vi "PID Table (Auto).vi"(6 "Ziegler-Nichlos Speed":u16(ring) items=["Fast", "Normal", "Slow"], 7 "Type of Controller":u16(ring) items=["P", "PI", "PID"], 8 "dT":dbl, 9 "Dead Time (L)":dbl, 10 "Time Constant (T)":dbl, 11 "Plant Gain (K)":dbl) -> (1 "Derivative Time (Td)":dbl, 2 "Integral Time (Ti)":dbl, 3 "Proportional Gain (Kp)":dbl)   [LabVIEW 2020, in "NI_PID_autopid.lvlib"]
uses:
  <vilib>/addons/control/pid/NI_PID_autopid.lvlib
  <vilib>/addons/control/pid/NI_PID_pid.lvlib
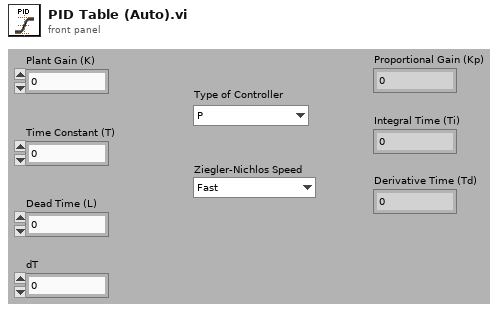
[diagram p1: front panel]
types:
  T1 = enum16{"Academic (Standard)", "Parallel", "Series"}
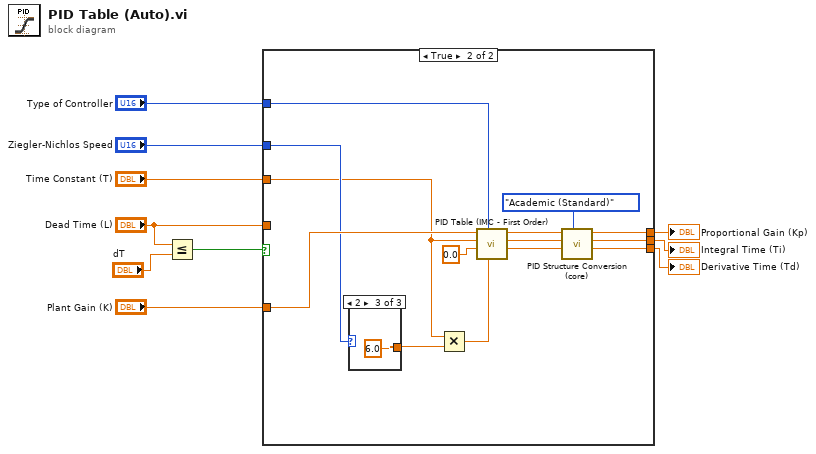
[diagram p0: block diagram]
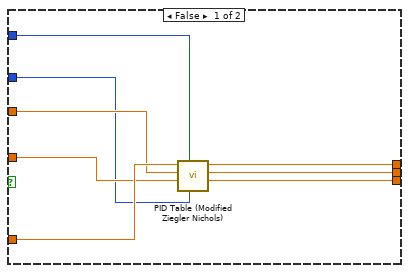
[diagram p2: hidden frame]
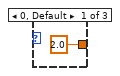
[diagram p3: hidden frame]
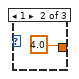
[diagram p4: hidden frame]
diagram:
  n1 = Less Or Equal?(x="Dead Time (L)", y="dT") -> (x <= y?=w1:bool)
  n2 = case shown="True" w1 {
    tunnel: "Plant Gain (K)" -> [w18 w32]
    tunnel: "Time Constant (T)" -> [w17 w27]
    tunnel: "Ziegler-Nichlos Speed" -> [w12 w28]
    tunnel: [w15 w25] -> w7
    tunnel: [w14 w23] -> w6
    tunnel: [w13 w21] -> w5
    tunnel: "Type of Controller" -> [w11 w30]
    tunnel: "Dead Time (L)" -> [w16 _]
    frame False {
      n3 = call <vilib>:"PID Table (Modified Ziegler Nichols).vi"("Ziegler-Nichlos Speed"=w12, "Type of Controller"=w11, "Dead Time (L)"=w16, "Time Constant (T)"=w17, "Plant Gain (K)"=w18) -> ("Derivative Time (Td)"=w13:dbl, "Integral Time (Ti)"=w14:dbl, "Proportional Gain (Kp)"=w15:dbl)  [unwired: 4 in]
    }
    frame True {
      n4 = case shown="2" w28 {
        tunnel: [2.0 ("y") 4.0 ("y") 6.0 ("y")] -> w29
        frame 0, Default {
        }
        frame 1 {
        }
        frame 2 {
        }
      }
      n5 = Multiply(x=w27, y=w29) -> (x*y=w19:dbl)
      n6 = call <vilib>:"PID Table (IMC - First Order).vi"("Desired Time Constant (tau_c)"=w19, "Type of Controller"=w30, "Plant delay (theta)"=0.0, "Plant time constant (tau)"=w27, "Plant gain (K)"=w32) -> ("TD"=w22:dbl, "Ti"=w24:dbl, "Kc"=w26:dbl)  [unwired: 4 in]
      n7 = call <vilib>:"PID Structure Conversion (core).vi"("PID structure"=T1."Academic (Standard)", "derivative in"=w22, "integral in"=w24, "proportional in"=w26) -> ("derivative time (s)"=w21:dbl, "integral time (s)"=w23:dbl, "proportional"=w25:dbl)  [unwired: 5 in]
    }
  }
  "Proportional Gain (Kp)" <- w7
  "Integral Time (Ti)" <- w6
  "Derivative Time (Td)" <- w5
